vi "Device Channel to Register Base Address.vi"(10 "Channel":i32 caption="通道") -> (2 "Register Base Address":u16 caption="寄存器基地址")   [LabVIEW 2023, in "Longer Pump dLSP501 Series.lvlib"]
uses:
  <instrlib>/Longer Pump dLSP501 Modbus RTU Series/Longer Pump dLSP501 Series.lvlib
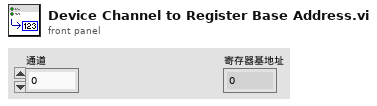
[diagram p1: front panel]
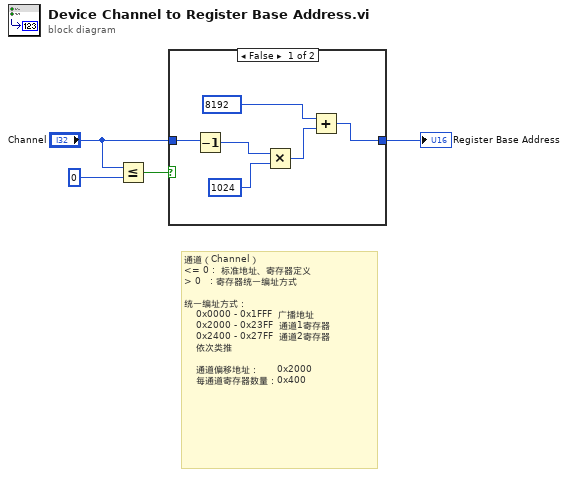
[diagram p0: block diagram]
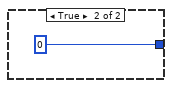
[diagram p2: hidden frame]
diagram:
  # "通道（Channel）\n<= 0 :  标准地址、寄存器定义\n> 0   : 寄存器统一编址方式\n\n统一编址方式：\n    0x0000 - 0x1FFF  广播地址\n    0x2000 - 0x23FF  通道1寄存器\n    0x2400 - 0x27FF  通道2寄存器\n    依次类推\n\n    通道偏移地址：      0x2000\n    每通道寄存器数量：0x400"
  n1 = Less Or Equal?(x="Channel", y=0) -> (x <= y?=w3:bool)
  n2 = case shown="False" w3 {
    tunnel: [w5 0 ("y")] -> w2
    tunnel: "Channel" -> [w9 _]
    frame False {
      n3 = Decrement(x=w9) -> (x-1=w10:i32)
      n4 = Multiply(x=w10, y=u16 1024) -> (x*y=w6:i32)
      n5 = Add(x=u16 8192 ("y"), y=w6) -> (x+y=w5:i32)
    }
    frame True {
    }
  }
  "Register Base Address" <- w2
